vi "CreatEditExcel v0.2.vi"(1 "output":dbl[][](array[numeric])) -> ()   [LabVIEW 2014]
panel:
  out "Excel._Application 2":refnum<k7>
  out "error out 2":errorcluster
  in  "Excel._Worksheet":refnum<k7>
  in  "error in":errorcluster
  in  "Excel._Application":refnum<k7>
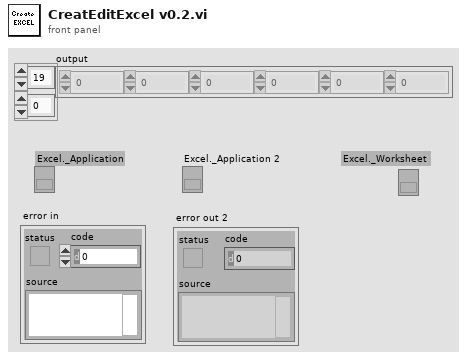
[diagram p1: front panel]
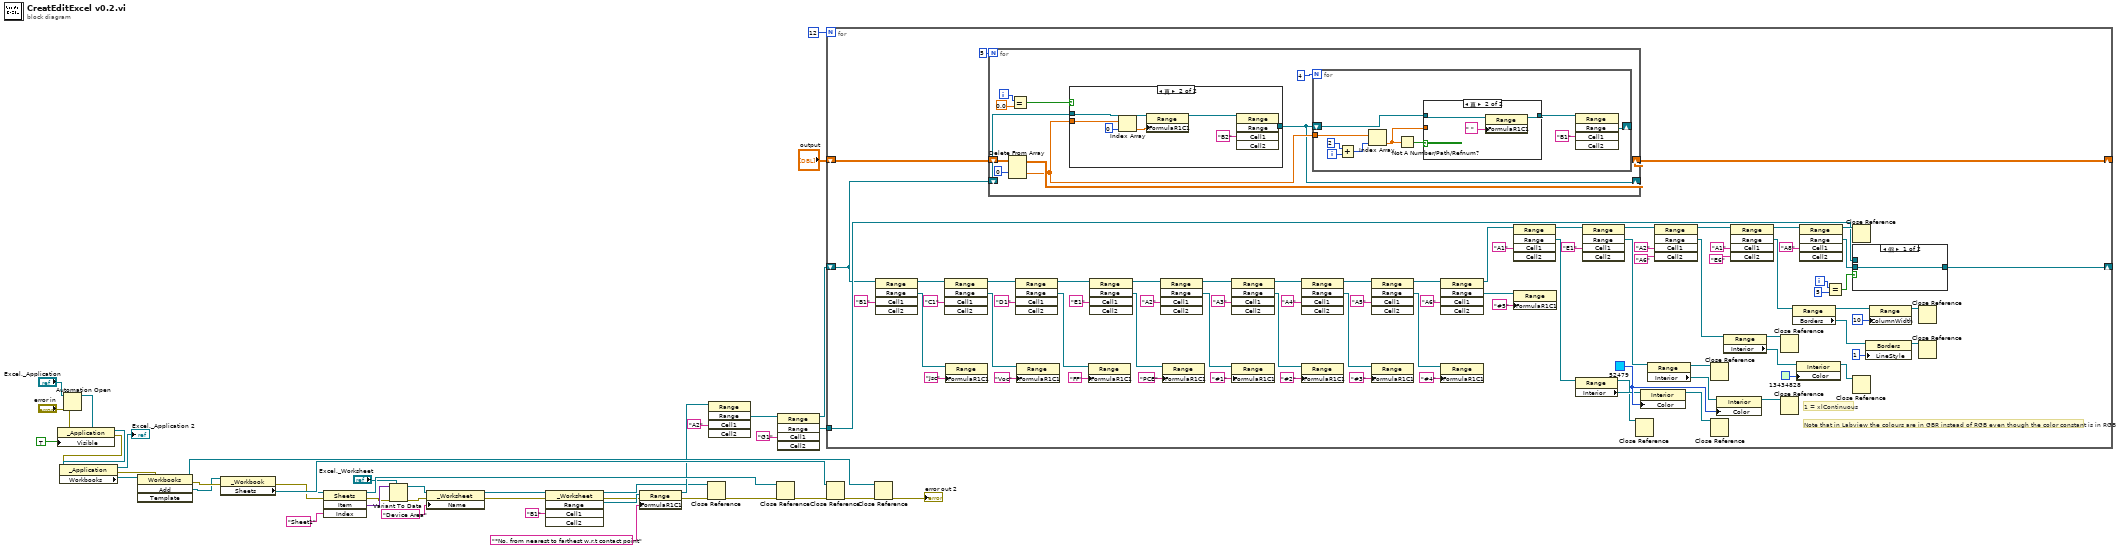
[diagram p0: block diagram]
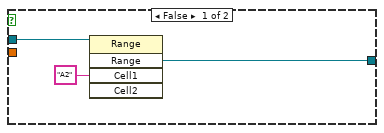
[diagram p2: hidden frame]
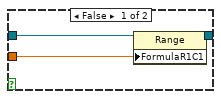
[diagram p3: hidden frame]
diagram:
  n1 = Automation Open(error in (no error)="error in", Automation Refnum="Excel._Application") -> (Automation Refnum=w43:refnum<k7>, error out=w44:errorcluster)  [unwired: 2 out]
  n2 = property class="_Application"(reference=w43, error in=w44, "Visible"=TRUE ("Visible Boolean")) -> (reference out=w37:refnum<k7>, error out=w36:errorcluster)
  n3 = property class="_Application"(reference=w37, error in=w36) -> (reference out=→"Excel._Application 2":refnum<k7>, error out=w38:errorcluster, "Workbooks"=w39:refnum<k7>)
  n4 = invoke class="Workbooks" method="Add"(reference=w39, error in=w38) -> (reference out=w30:refnum<k7>, error out=w34:errorcluster, "Add"=w1:refnum<k7>)  [unwired: 2 in, 1 out]
  n5 = property class="_Workbook"(reference=w1, error in=w34) -> (reference out=w26:refnum<k7>, error out=w15:errorcluster, "Sheets"=w20:refnum<k7>)
  n6 = invoke class="Sheets" method="Item"(reference=w20, error in=w15, "Index"="Sheet1") -> (reference out=w27:refnum<k7>, error out=w32:errorcluster, "Item"=w35:variant)  [unwired: 1 in, 1 out]
  n7 = Variant To Data(error in=w32, type="Excel._Worksheet", Variant=w35) -> (data=w19:refnum<k7>, error out=w13:errorcluster)
  n8 = property class="_Worksheet"(reference=w19, error in=w13, "Name"="Device Area") -> (reference out=w18:refnum<k7>, error out=w17:errorcluster)
  n9 = invoke class="_Worksheet" method="Range"(reference=w18, error in=w17, "Cell1"="B1") -> (reference out=w3:refnum<k7>, error out=w22:errorcluster, "Range"=w24:refnum<k7>)  [unwired: 2 in, 2 out]
  n10 = property class="Range"(reference=w24, error in=w22, "FormulaR1C1"="*No. from nearest to farthest w.r.t contact point") -> (reference out=w12:refnum<k7>, error out=w4:errorcluster)
  n11 = Close Reference(reference=w3, error in (no error)=w4) -> (error out=w2:errorcluster)
  n12 = invoke class="Range" method="Range"(reference=w12, "Cell1"="A2") -> ("Range"=w9:refnum<k7>)  [unwired: 3 in, 4 out]
  n13 = Close Reference(reference=w27, error in (no error)=w2) -> (error out=w31:errorcluster)
  n14 = invoke class="Range" method="Range"(reference=w9, "Cell1"="G1") -> (reference out=w6:refnum<k7>, "Range"=w7:refnum<k7>)  [unwired: 3 in, 3 out]
  n15 = for {
    N: 12 -> [_]
    shift-right: [w50] -> _
    shift-left: w6 -> [w45]
    tunnel: w7 -> [w51]
    shift-right: [w46] -> _
    shift-left: "output" -> [w47]
    i -> [w52]
    w97 = u32 52479
    # "1 = xlContinuous"
    # "Note that in Labview the colours are in GBR instead of RGB even though the color constant is in RGB"
    n16 = invoke class="Range" method="Range"(reference=w45, "Cell1"="B1") -> (reference out=w71:refnum<k7>, "Range"=w72:refnum<k7>)  [unwired: 3 in, 3 out]
    n17 = invoke class="Range" method="Range"(reference=w71, "Cell1"="C1") -> (reference out=w69:refnum<k7>, "Range"=w70:refnum<k7>)  [unwired: 3 in, 3 out]
    n18 = property class="Range"(reference=w72, "FormulaR1C1"="Jsc") -> ()  [unwired: 1 in, 2 out]
    n19 = for {
      N: 5 -> [_]
      shift-right: [w132] -> w46
      shift-left: w47 -> [w133]
      shift-right: [w124] -> _
      shift-left: w45 -> [w126]
      i -> [w128]
      n20 = Delete From Array(array=w133, index (row)=0) -> (deleted portion=w125:dbl[], array with subset deleted=w132:dbl[][])  [unwired: 2 in]
      n21 = Equal?(x=w128, y=0.0) -> (x = y?=w127:bool)
      n22 = case shown="真" w127 {
        tunnel: [w134 w143] -> w124
        tunnel: w126 -> [w135 w138]
        tunnel: w125 -> [_ w139]
        frame False {
          n23 = invoke class="Range" method="Range"(reference=w135, "Cell1"="A2") -> ("Range"=w134:refnum<k7>)  [unwired: 3 in, 4 out]
        }
        frame True {
          n24 = Index Array(array=w139, index=0) -> (element=w140:dbl)
          n25 = property class="Range"(reference=w138, "FormulaR1C1"=w140) -> (reference out=w137:refnum<k7>)  [unwired: 1 in, 1 out]
          n26 = invoke class="Range" method="Range"(reference=w137, "Cell1"="B2") -> ("Range"=w143:refnum<k7>)  [unwired: 3 in, 4 out]
        }
      }
      n27 = for {
        N: 4 -> [_]
        tunnel: w125 -> [w150]
        shift-right: [w148] -> _
        shift-left: w124 -> [w145]
        i -> [w153]
        n28 = Add(x=2, y=w153) -> (x+y=w151:i32)
        n29 = Index Array(array=w150, index=w151) -> (element=w146:dbl)
        n30 = Not A Number/Path/Refnum?(number/path/refnum=w146) -> (NaN/Path/Refnum?=w147:bool)
        n31 = case shown="真" w147 {
          tunnel: w146 -> [w155 _]
          tunnel: w145 -> [w156 w158]
          tunnel: [w154 w159] -> w144
          frame False {
            n32 = property class="Range"(reference=w156, "FormulaR1C1"=w155) -> (reference out=w154:refnum<k7>)  [unwired: 1 in, 1 out]
          }
          frame True {
            n33 = property class="Range"(reference=w158, "FormulaR1C1"=" ") -> (reference out=w159:refnum<k7>)  [unwired: 1 in, 1 out]
          }
        }
        n34 = invoke class="Range" method="Range"(reference=w144, "Cell1"="B1") -> ("Range"=w148:refnum<k7>)  [unwired: 3 in, 4 out]
      }
    }
    n35 = invoke class="Range" method="Range"(reference=w69, "Cell1"="D1") -> (reference out=w67:refnum<k7>, "Range"=w68:refnum<k7>)  [unwired: 3 in, 3 out]
    n36 = property class="Range"(reference=w70, "FormulaR1C1"="Voc") -> ()  [unwired: 1 in, 2 out]
    n37 = property class="Range"(reference=w68, "FormulaR1C1"="FF") -> ()  [unwired: 1 in, 2 out]
    n38 = invoke class="Range" method="Range"(reference=w67, "Cell1"="E1") -> (reference out=w55:refnum<k7>, "Range"=w66:refnum<k7>)  [unwired: 3 in, 3 out]
    n39 = invoke class="Range" method="Range"(reference=w55, "Cell1"="A2") -> (reference out=w64:refnum<k7>, "Range"=w65:refnum<k7>)  [unwired: 3 in, 3 out]
    n40 = property class="Range"(reference=w66, "FormulaR1C1"="PCE") -> ()  [unwired: 1 in, 2 out]
    n41 = invoke class="Range" method="Range"(reference=w64, "Cell1"="A3") -> (reference out=w62:refnum<k7>, "Range"=w63:refnum<k7>)  [unwired: 3 in, 3 out]
    n42 = property class="Range"(reference=w65, "FormulaR1C1"="#1") -> ()  [unwired: 1 in, 2 out]
    n43 = invoke class="Range" method="Range"(reference=w62, "Cell1"="A4") -> (reference out=w60:refnum<k7>, "Range"=w61:refnum<k7>)  [unwired: 3 in, 3 out]
    n44 = property class="Range"(reference=w63, "FormulaR1C1"="#2") -> ()  [unwired: 1 in, 2 out]
    n45 = invoke class="Range" method="Range"(reference=w60, "Cell1"="A5") -> (reference out=w58:refnum<k7>, "Range"=w59:refnum<k7>)  [unwired: 3 in, 3 out]
    n46 = property class="Range"(reference=w61, "FormulaR1C1"="#3") -> ()  [unwired: 1 in, 2 out]
    n47 = invoke class="Range" method="Range"(reference=w58, "Cell1"="A6") -> (reference out=w56:refnum<k7>, "Range"=w57:refnum<k7>)  [unwired: 3 in, 3 out]
    n48 = property class="Range"(reference=w59, "FormulaR1C1"="#4") -> ()  [unwired: 1 in, 2 out]
    n49 = invoke class="Range" method="Range"(reference=w56, "Cell1"="A1") -> (reference out=w87:refnum<k7>, "Range"=w88:refnum<k7>)  [unwired: 3 in, 3 out]
    n50 = property class="Range"(reference=w57, "FormulaR1C1"="#5") -> ()  [unwired: 1 in, 2 out]
    n51 = property class="Range"(reference=w88) -> (reference out=w78:refnum<k7>, "Interior"=w89:refnum<k7>)  [unwired: 1 in, 1 out]
    n52 = invoke class="Range" method="Range"(reference=w87, "Cell1"="E1") -> (reference out=w86:refnum<k7>, "Range"=w95:refnum<k7>)  [unwired: 3 in, 3 out]
    n53 = Close Reference(reference=w78) -> ()  [unwired: 1 in, 1 out]
    n54 = property class="Interior"(reference=w89, "Color"=w97) -> (reference out=w77:refnum<k7>)  [unwired: 1 in, 1 out]
    n55 = property class="Range"(reference=w95) -> (reference out=w79:refnum<k7>, "Interior"=w96:refnum<k7>)  [unwired: 1 in, 1 out]
    n56 = invoke class="Range" method="Range"(reference=w86, "Cell1"="A2", "Cell2"="A6") -> (reference out=w85:refnum<k7>, "Range"=w92:refnum<k7>)  [unwired: 2 in, 3 out]
    n57 = Close Reference(reference=w79) -> ()  [unwired: 1 in, 1 out]
    n58 = Close Reference(reference=w77) -> ()  [unwired: 1 in, 1 out]
    n59 = property class="Interior"(reference=w96, "Color"=w97) -> (reference out=w76:refnum<k7>)  [unwired: 1 in, 1 out]
    n60 = property class="Range"(reference=w92) -> (reference out=w80:refnum<k7>, "Interior"=w93:refnum<k7>)  [unwired: 1 in, 1 out]
    n61 = invoke class="Range" method="Range"(reference=w85, "Cell1"="A1", "Cell2"="E6") -> (reference out=w75:refnum<k7>, "Range"=w98:refnum<k7>)  [unwired: 2 in, 3 out]
    n62 = Close Reference(reference=w80) -> ()  [unwired: 1 in, 1 out]
    n63 = Close Reference(reference=w76) -> ()  [unwired: 1 in, 1 out]
    n64 = property class="Range"(reference=w98) -> (reference out=w84:refnum<k7>, "Borders"=w90:refnum<k7>)  [unwired: 1 in, 1 out]
    n65 = property class="Interior"(reference=w93, "Color"=u32 13434828) -> (reference out=w81:refnum<k7>)  [unwired: 1 in, 1 out]
    n66 = invoke class="Range" method="Range"(reference=w75, "Cell1"="A8") -> (reference out=w73:refnum<k7>, "Range"=w49:refnum<k7>)  [unwired: 3 in, 3 out]
    n67 = Equal?(x=w52, y=5) -> (x = y?=w53:bool)
    n68 = Close Reference(reference=w73) -> ()  [unwired: 1 in, 1 out]
    n69 = case shown="假" w53 {
      tunnel: w51 -> [_ w161]
      tunnel: [w160 w161] -> w50
      tunnel: w49 -> [w160 _]
      frame False {
      }
      frame True {
      }
    }
    n70 = Close Reference(reference=w81) -> ()  [unwired: 1 in, 1 out]
    n71 = property class="Borders"(reference=w90, "LineStyle"=1 ("Row Offset")) -> (reference out=w82:refnum<k7>)  [unwired: 1 in, 1 out]
    n72 = property class="Range"(reference=w84, "ColumnWidth"=10 ("Row Offset")) -> (reference out=w83:refnum<k7>)  [unwired: 1 in, 1 out]
    n73 = Close Reference(reference=w83) -> ()  [unwired: 1 in, 1 out]
    n74 = Close Reference(reference=w82) -> ()  [unwired: 1 in, 1 out]
  }
  n75 = Close Reference(reference=w26, error in (no error)=w31) -> (error out=w29:errorcluster)
  n76 = Close Reference(reference=w30, error in (no error)=w29) -> (error out=→"error out 2":errorcluster)
